vi "Compiler Tree Structure.VI"(0 "Tree formula":T1(array[cluster])) -> (1 "Result":dbl[](array[numeric]) format="%0.2f", 2 "Table":i32[][](array[numeric]))   [LabVIEW 2020, in "NI_Gmath.lvlib"]
uses:
  NI_Gmath.lvlib
panel:
  # "operator"
  # "register1"
  # "register2"
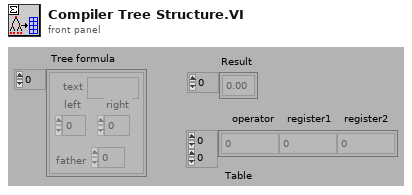
[diagram p1: front panel]
types:
  T1 = cluster{"text":string, "left":i32, "right":i32, "father":i32}[]
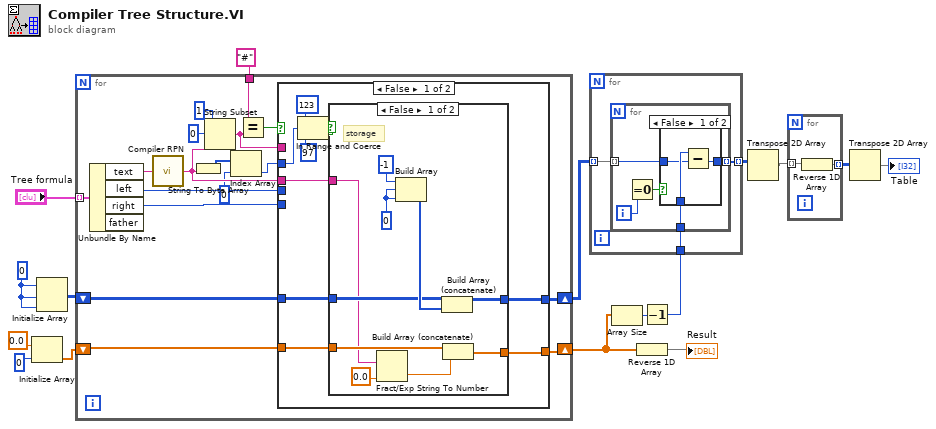
[diagram p0: block diagram]
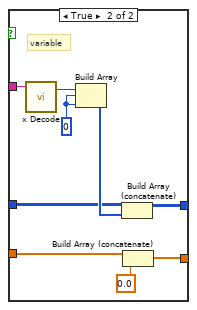
[diagram p3: hidden frame]
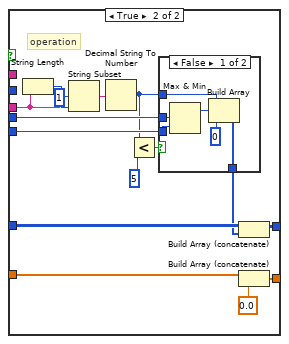
[diagram p4: hidden frame]
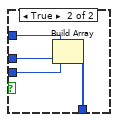
[diagram p5: hidden frame]
diagram:
  w14 = 0
  n1 = Initialize Array(0.0, 0) -> (w10:dbl[])
  n2 = Initialize Array(w14, w14, w14) -> (w13:i32[][])
  n3 = for {
    tunnel: "Tree formula" -> [w33] mode=indexing
    tunnel: "#" -> [w29]
    shift-right: [w24] -> w8
    shift-left: w13 -> [w25]
    shift-right: [w21] -> w3
    shift-left: w10 -> [w22]
    n4 = Unbundle By Name(w33) -> ("text"=w32:string, "left"=w27:i32, "right"=w26:i32)  [unwired: 1 out]
    n5 = call "Compiler RPN.VI"("string"=w32) -> ("result as string"=w20:string)
    n6 = String To Byte Array(string=w20) -> (unsigned byte array=w19:u8[])
    n7 = String Subset(string=w20, offset (0)=0, length (rest)=1) -> (substring=w23:string)
    n8 = Index Array(array=w19, index=0) -> (element=w17:u8)
    n9 = Equal?(x=w29, y=w23) -> (x = y?=w28:bool)
    n10 = case shown="False" w28 {
      tunnel: w20 -> [w42 w68]
      tunnel: w27 -> [_ w65]
      tunnel: w26 -> [_ w66]
      tunnel: w25 -> [w41 w74]
      tunnel: [w40 w72] -> w24
      tunnel: w23 -> [_ _]
      tunnel: w22 -> [w39 w71]
      tunnel: [w38 w69] -> w21
      tunnel: w17 -> [w37 _]
      frame False {
        n11 = In Range and Coerce(upper limit=123, x=w37, lower limit=97) -> (In Range?=w34:bool)  [unwired: 1 out]
        n12 = case shown="False" w34 {
          tunnel: w42 -> [w45 w54]
          tunnel: w41 -> [w50 w59]
          tunnel: [w49 w58] -> w40
          tunnel: w39 -> [w47 w56]
          tunnel: [w46 w55] -> w38
          frame False {
            w52 = 0
            # "storage"
            n13 = Fract/Exp String To Number(string=w45, default (0 dbl)=0.0) -> (number=w44:dbl)  [unwired: 2 in, 1 out]
            n14 = Build Array(-1, w52, w52) -> (w51:i32[])
            n15 = Build Array (concatenate)(w50, w51) -> (w49:i32[][])
            n16 = Build Array (concatenate)(w47, w44) -> (w46:dbl[])
          }
          frame True {
            w61 = 0
            # "variable"
            n17 = call "x Decode.vi"("x string"=w54) -> ("number"=w53:i32)  [unwired: 1 in, 1 out]
            n18 = Build Array(w53, w61, w61) -> (w60:i32[])
            n19 = Build Array (concatenate)(w59, w60) -> (w58:i32[][])
            n20 = Build Array (concatenate)(w56, 0.0) -> (w55:dbl[])
          }
        }
      }
      frame True {
        # "operation"
        n21 = String Length(string=w68) -> (length=w76:i32)
        n22 = String Subset(string=w68, offset (0)=1, length (rest)=w76) -> (substring=w67:string)
        n23 = Decimal String To Number(string=w67) -> (number=w64:i32)  [unwired: 2 in, 1 out]
        n24 = Less?(x=w64, y=5) -> (x < y?=w62:bool)
        n25 = case shown="False" w62 {
          tunnel: w65 -> [w80 w86]
          tunnel: w66 -> [w79 w85]
          tunnel: w64 -> [w82 w84]
          tunnel: [w81 w83] -> w73
          frame False {
            n26 = Max & Min(x=w80, y=w79) -> (max(x,y)=w78:i32)  [unwired: 1 out]
            n27 = Build Array(w82, w78, 0) -> (w81:i32[])
          }
          frame True {
            n28 = Build Array(w84, w86, w85) -> (w83:i32[])
          }
        }
        n29 = Build Array (concatenate)(w74, w73) -> (w72:i32[][])
        n30 = Build Array (concatenate)(w71, 0.0) -> (w69:dbl[])
      }
    }
  }
  n31 = Array Size(array=w3) -> (size(s)=w9:i32)
  n32 = Reverse 1D Array(array=w3) -> (reversed array=→"Result":dbl[])
  n33 = Decrement(x=w9) -> (x-1=w7:i32)
  n34 = for {
    tunnel: w8 -> [w89] mode=indexing
    tunnel: [w88] -> w4 mode=indexing
    tunnel: w7 -> [w87]
    n35 = for {
      tunnel: w89 -> [w92] mode=indexing
      tunnel: [w91] -> w88 mode=indexing
      tunnel: w87 -> [w90]
      i -> [w94]
      n36 = Equal To 0?(x=w94) -> (x = 0?=w93:bool)
      n37 = case shown="False" w93 {
        tunnel: [w95 w98] -> w91
        tunnel: w92 -> [w96 w98]
        tunnel: w90 -> [w97 _]
        frame False {
          n38 = Subtract(x=w97, y=w96) -> (x-y=w95:i32)
        }
        frame True {
        }
      }
    }
  }
  n39 = Transpose 2D Array(2D array=w4) -> (transposed array=w6:i32[][])
  n40 = for {
    tunnel: w6 -> [w100] mode=indexing
    tunnel: [w99] -> w5 mode=indexing
    n41 = Reverse 1D Array(array=w100) -> (reversed array=w99:i32[])
  }
  n42 = Transpose 2D Array(2D array=w5) -> (transposed array=→"Table":i32[][])
